vi "PUT Power Peak.vi"(0 "Power Peak":dbl) -> ()   [LabVIEW 2013]
uses:
  Action.ctl
  Calibration Output FGV Selector.ctl
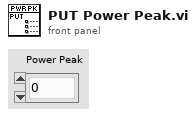
[diagram p1: front panel]
types:
  T1 = typedef "Calibration Output FGV Selector.ctl" = enum16{"Power Peak", "Slope", "Spring Constant"}
  T2 = typedef "Action.ctl" = enum16{"GET", "PUT", "DELETE"}
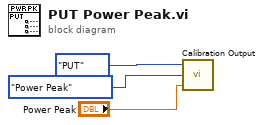
[diagram p0: block diagram]
diagram:
  n1 = call "Calibration Output.vi"("Input"="Power Peak", "Calibration Output FGV Selector"=Calibration_Output_FGV_Selector."Power Peak", "Action"=Action."PUT") -> ()  [unwired: 1 out]
